vi "AI Array Add or Remove.vi"(8 "error in (no error)":errorcluster, 10 "Size":i32, 11 "AI Channels":T1[](array[typedef]) {"References" items=["", "1", "2", "3"]}) -> (0 "error out":errorcluster, 3 "AI Channels out":T1[](array[typedef]) {"References" items=["", "1", "2", "3"]})   [LabVIEW 2016, in "Instrument.Lockin.lvclass"]
uses:
  Instrument.Lockin.lvclass
  Instrument.Lockinl.UI/Typedefs/AI Channel--Cluster.ctl
  Instrument.Lockinl.UI/Instrument.Lockin.UI.lvclass
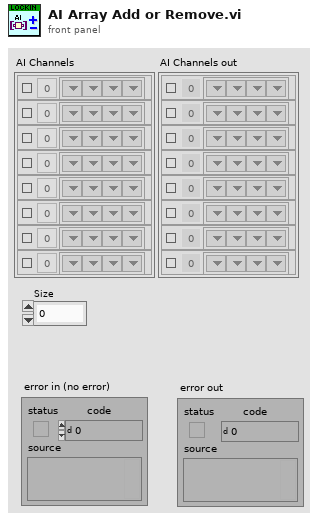
[diagram p1: front panel]
types:
  T1 = typedef "Instrument.Lockin.UI.lvclass/AI Channel--Cluster.ctl" = cluster{"Enable?":bool, "Channel":i32, "References":u16[]}
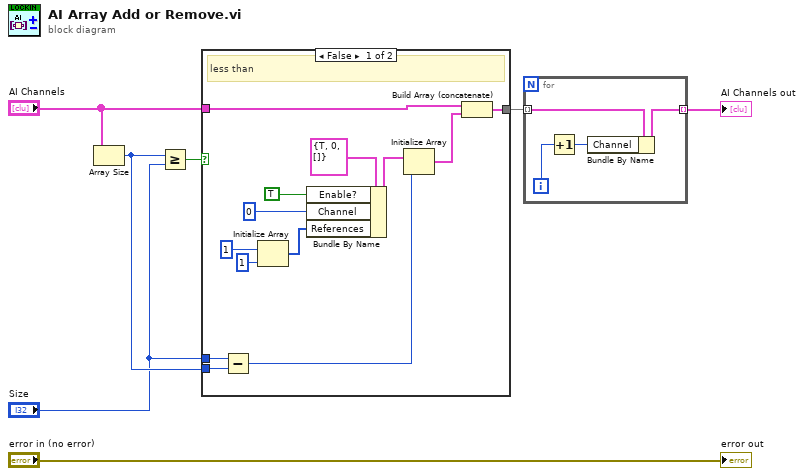
[diagram p0: block diagram]
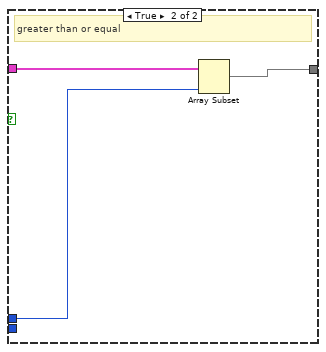
[diagram p2: hidden frame]
diagram:
  n1 = Array Size(array="AI Channels") -> (size(s)=w7:i32)
  n2 = Greater Or Equal?(x=w7, y="Size") -> (x >= y?=w6:bool)
  n3 = case shown="False" w6 {
    tunnel: "AI Channels" -> [w15 w23]
    tunnel: "Size" -> [w18 w22]
    tunnel: [w19 w21] -> w3
    tunnel: w7 -> [w17 _]
    frame False {
      # "less than"
      n4 = Subtract(x=w18, y=w17) -> (x-y=w16:i32)
      n5 = Initialize Array(u16 1 ("Reference 1"), 1 ("dimension size")) -> (w8:u16[])
      n6 = Bundle By Name(cluster=T1 {"Enable?"=TRUE, "Channel"=0, "References"=[]} ("AO"), "Enable?"=TRUE, "Channel"=0, "References"=w8) -> (w13:T1)
      n7 = Initialize Array(w13, w16) -> (w20:T1[])
      n8 = Build Array (concatenate)(w15, w20) -> (w19:T1[])
    }
    frame True {
      # "greater than or equal"
      n9 = Array Subset(array=w23, length=w22) -> (w21:T1[])  [unwired: 1 in]
    }
  }
  n10 = for {
    tunnel: w3 -> [w27] mode=indexing
    tunnel: [w26] -> w2 mode=indexing
    i -> [w24]
    n11 = Increment(x=w24) -> (x+1=w25:i32)
    n12 = Bundle By Name(cluster=w27, "Channel"=w25) -> (w26:T1)
  }
  "AI Channels out" <- w2
  "error out" <- "error in (no error)"
